vi "Performance.vi"() -> ()   [LabVIEW 2011]
uses:
  fg_typedef.ctl
  <vilib>/NI_Real-Time Target Support.lvlib
panel:
  in  "Boolean 2":bool
  in  "Boolean":bool
  out "Total CPU (%)":dbl
  out "RAM available (bytes)":u32
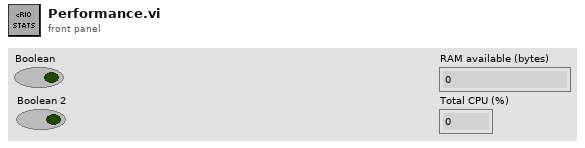
[diagram p1: front panel]
types:
  T1 = typedef "fg_typedef.ctl" = enum16{"Get", "Set"}
  T2 = typedef "NI_Real-Time Target Support.lvlib/RT CPU Load.ctl" = cluster{"Total (%)":dbl, "Time Critical (%)":dbl, "Timed Structures (%)":dbl, "High (%)":dbl, "Above Normal (%)":dbl, "Normal (%)":dbl, "Background (%)":dbl, "Idle (%)":dbl, "ISR (%)":dbl}
  T3 = cluster{"CPU Usage":dbl, "RAM Available":u32, "Vision mSPI":u32, "Main mSPI":u32}
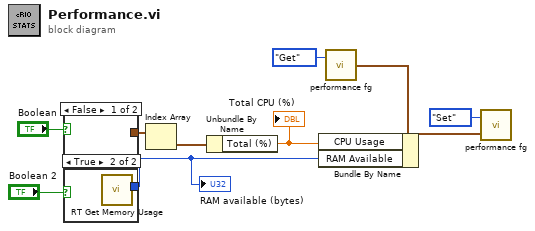
[diagram p0: block diagram]
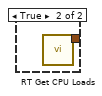
[diagram p3: hidden frame]
diagram:
  n1 = case shown="False" "Boolean" {
    tunnel: [_ w11] -> w10
    frame False {
    }
    frame True {
      n2 = call <vilib>:"RT Get CPU Loads.vi"() -> ("CPU loads"=w11:T2[])  [unwired: 10 in, 1 out]
    }
  }
  n3 = case shown="True" "Boolean 2" {
    tunnel: [_ w12] -> w7
    frame False {
    }
    frame True {
      n4 = call <vilib>:"RT Get Memory Usage.vi"() -> ("available (bytes)"=w12:u32)  [unwired: 8 in, 3 out]
    }
  }
  "RAM available (bytes)" <- w7
  n5 = Index Array(array=w10) -> (element=w9:T2)  [unwired: 1 in]
  n6 = Unbundle By Name(w9) -> ("Total (%)"=w8:dbl)
  "Total CPU (%)" <- w8
  n7 = call "performance fg.vi"("Menu"=fg_typedef."Get") -> ("Output"=w3:T3)  [unwired: 1 in]
  n8 = Bundle By Name(cluster=w3, "CPU Usage"=w8, "RAM Available"=w7) -> (w5:T3)
  n9 = call "performance fg.vi"("Input"=w5, "Menu"=fg_typedef."Set") -> ()  [unwired: 1 out]
